vi "mono_camera_array_display.vi"(3 "error in (no error)":errorcluster, 5 "camera connections input":T2, 6 "camera dimensions input":T3) -> (0 "connections out":T4, 1 "camera array out":T1)   [LabVIEW 2018, in "monoDrive.lvlib"]
uses:
  monoDrive.lvlib
panel:
  in  "camera array def":T1
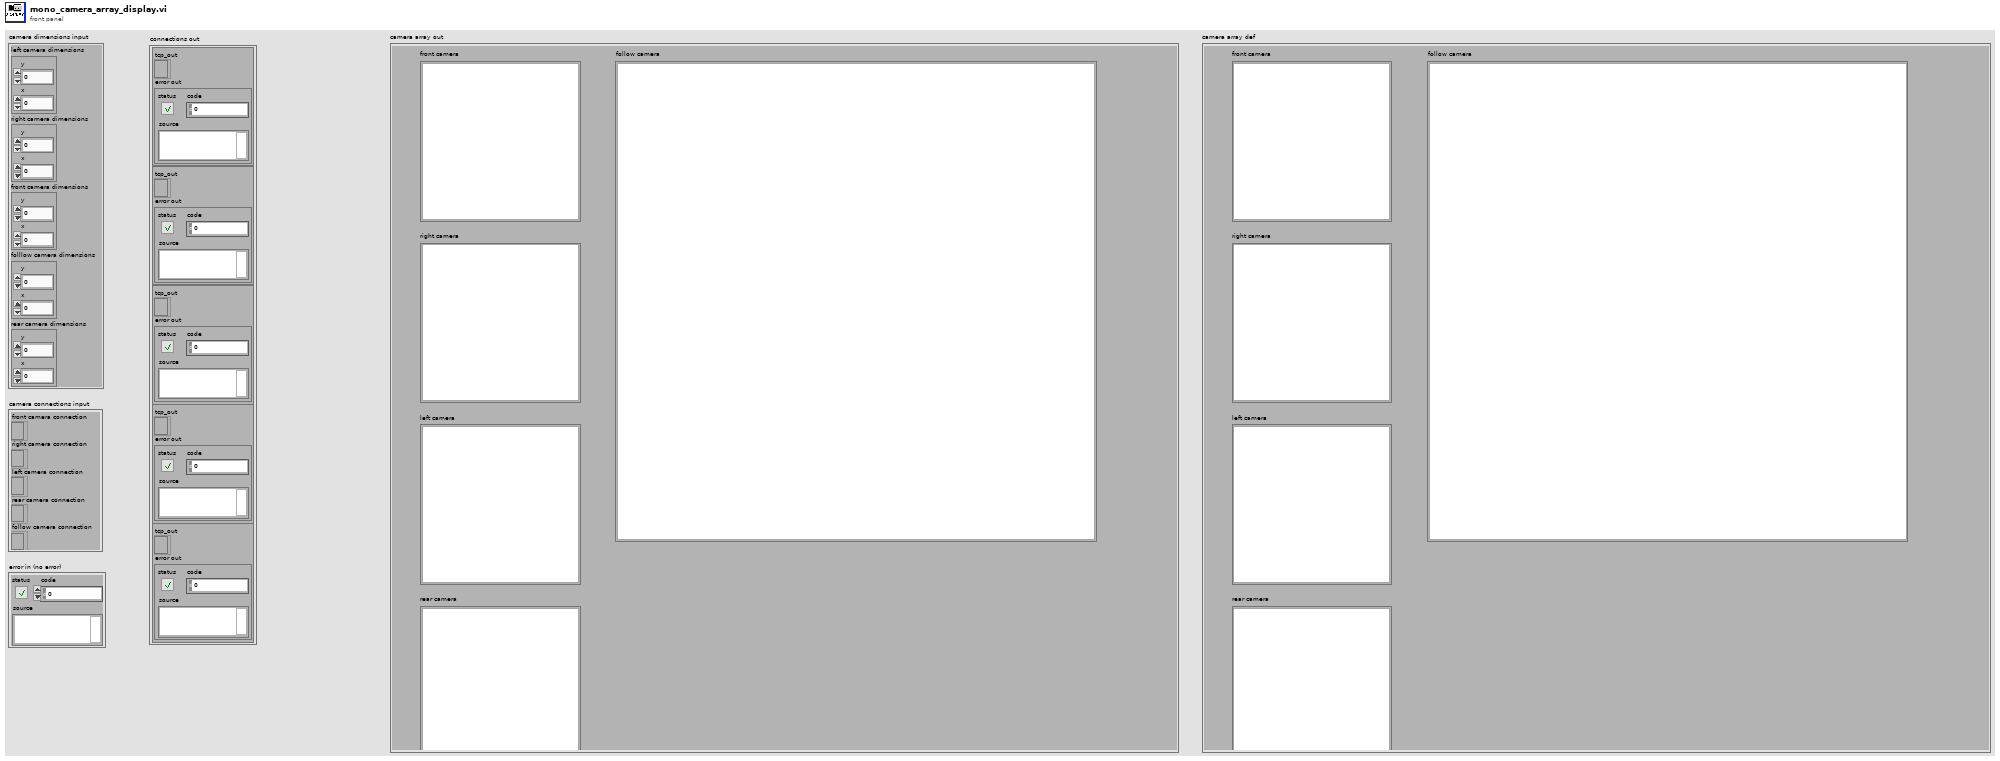
[diagram p1: front panel]
types:
  T1 = cluster{"follow camera":picture, "rear camera":picture, "left camera":picture, "right camera":picture, "front camera":picture}
  T2 = cluster{"front camera connection":refnum<k5>, "right camera connection":refnum<k5>, "left camera connection":refnum<k5>, "rear camera connection":refnum<k5>, "follow camera connection":refnum<k5>}
  T3 = cluster{"left camera dimensions":cluster{"y ":i32, "x ":i32}, "right camera dimensions":cluster{"y":i32, "x":i32}, "front camera dimensions":cluster{"y":i32, "x":i32}, "folllow camera dimensions":cluster{"y":i32, "x":i32}, "rear camera dimensions":cluster{"y":i32, "x ":i32}}
  T4 = cluster{cluster{"tcp_out":refnum<k5>, "error out":errorcluster}, cluster{"tcp_out":refnum<k5>, "error out":errorcluster}, cluster{"tcp_out":refnum<k5>, "error out":errorcluster}, cluster{"tcp_out":refnum<k5>, "error out":errorcluster}, cluster{"tcp_out":refnum<k5>, "error out":errorcluster}}
  T5 = cluster{"tcp_out":refnum<k5>, "error out":errorcluster}
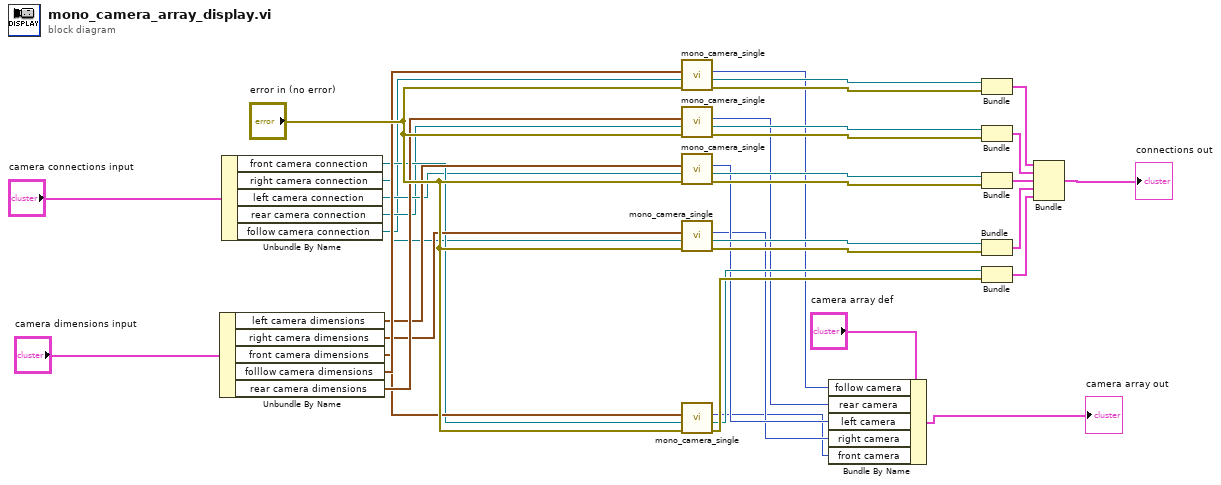
[diagram p0: block diagram]
diagram:
  n1 = Unbundle By Name("camera dimensions input") -> ("left camera dimensions"=w13:cluster{"y ":i32, "x ":i32}, "right camera dimensions"=w14:cluster{"y":i32, "x":i32}, "front camera dimensions"=w15:cluster{"y":i32, "x":i32}, "folllow camera dimensions"=w17:cluster{"y":i32, "x":i32}, "rear camera dimensions"=w16:cluster{"y":i32, "x ":i32})
  n2 = Unbundle By Name("camera connections input") -> ("front camera connection"=w12:refnum<k5>, "right camera connection"=w11:refnum<k5>, "left camera connection"=w10:refnum<k5>, "rear camera connection"=w9:refnum<k5>, "follow camera connection"=w8:refnum<k5>)
  n3 = call "mono_camera_single.vi"("error in"="error in (no error)", "connection ID"=w8, "stream dimensions"=w17) -> ("error out"=w22:errorcluster, "tcp_out"=w21:refnum<k5>, "camera_out"=w6:picture)  [unwired: 2 in]
  n4 = call "mono_camera_single.vi"("error in"="error in (no error)", "connection ID"=w9, "stream dimensions"=w16) -> ("error out"=w25:errorcluster, "tcp_out"=w24:refnum<k5>, "camera_out"=w5:picture)  [unwired: 2 in]
  n5 = call "mono_camera_single.vi"("error in"="error in (no error)", "connection ID"=w10, "stream dimensions"=w13) -> ("error out"=w28:errorcluster, "tcp_out"=w27:refnum<k5>, "camera_out"=w4:picture)  [unwired: 2 in]
  n6 = call "mono_camera_single.vi"("error in"="error in (no error)", "connection ID"=w11, "stream dimensions"=w14) -> ("error out"=w31:errorcluster, "tcp_out"=w30:refnum<k5>, "camera_out"=w3:picture)  [unwired: 2 in]
  n7 = call "mono_camera_single.vi"("error in"="error in (no error)", "connection ID"=w12, "stream dimensions"=w15) -> ("error out"=w33:errorcluster, "tcp_out"=w32:refnum<k5>, "camera_out"=w2:picture)  [unwired: 2 in]
  n8 = Bundle By Name(cluster="camera array def", "follow camera"=w6, "rear camera"=w5, "left camera"=w4, "right camera"=w3, "front camera"=w2) -> (→"camera array out":T1)
  n9 = Bundle("tcp_out"=w21, "error out"=w22) -> (w23:T5)  [unwired: 1 in]
  n10 = Bundle("tcp_out"=w24, "error out"=w25) -> (w26:T5)  [unwired: 1 in]
  n11 = Bundle("tcp_out"=w27, "error out"=w28) -> (w29:T5)  [unwired: 1 in]
  n12 = Bundle("tcp_out"=w30, "error out"=w31) -> (w34:T5)  [unwired: 1 in]
  n13 = Bundle("tcp_out"=w32, "error out"=w33) -> (w35:T5)  [unwired: 1 in]
  n14 = Bundle(w23, w26, w29, w34, w35) -> (→"connections out":T4)  [unwired: 1 in]
